vi "Get All Channels.vi"(7 "GUID (Default Channel)":string="03D3BB99-1485-13A6-561D1F898F032919", 8 "error in (no error)":errorcluster, 11 "Item Ref in":T1 format="%.0x") -> (0 "error out":errorcluster, 2 "Channels refs":T1[](array[typedef]) format="%.0x", 3 "Item Ref out":T1 format="%.0x")   [LabVIEW 2017, in "DSF Shared.lvlib"]
uses:
  DSF Shared.lvlib
  <vilib>/NI Veristand/Custom Device API/Custom Device Item Ref.ctl
  <vilib>/NI Veristand/Custom Device API/Custom Device API.lvlib
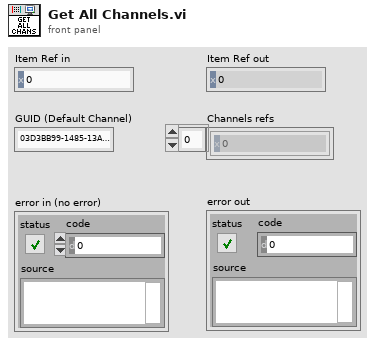
[diagram p1: front panel]
types:
  T1 = typedef "Custom Device API.lvlib/Custom Device Item Ref.ctl" = u64
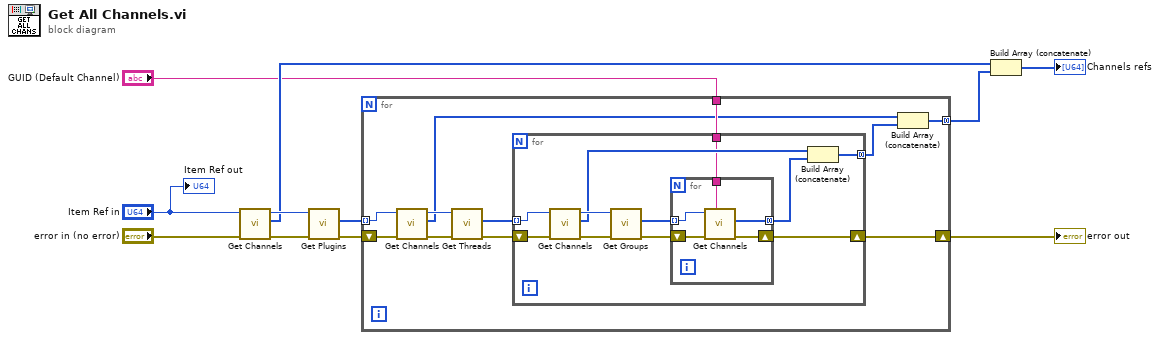
[diagram p0: block diagram]
diagram:
  n1 = call "Get Channels.vi"("error in (no error)"="error in (no error)", "Item Ref in"="Item Ref in") -> ("error out"=w6:errorcluster, "Channels refs"=w3:T1[], "Item Ref out"=w5:T1)  [unwired: 7 in]
  n2 = call "Get Plugins.vi"("error in (no error)"=w6, "Item Ref in"=w5) -> ("error out"=w11:errorcluster, "Plugin refs"=w10:T1[])  [unwired: 7 in, 1 out]
  n3 = for {
    tunnel: w10 -> [w19] mode=indexing
    tunnel: [w12] -> w8 mode=concatenating
    tunnel: "GUID (Default Channel)" -> [w21]
    shift-right: [w22] -> w2
    shift-left: w11 -> [w20]
    n4 = call "Get Channels.vi"("error in (no error)"=w20, "Item Ref in"=w19) -> ("error out"=w18:errorcluster, "Channels refs"=w13:T1[], "Item Ref out"=w17:T1)  [unwired: 7 in]
    n5 = call "Get Threads.vi"("error in (no error)"=w18, "Item Ref in"=w17) -> ("error out"=w16:errorcluster, "Plugin refs"=w15:T1[])  [unwired: 7 in, 1 out]
    n6 = for {
      shift-right: [w24] -> w22
      shift-left: w16 -> [w29]
      tunnel: w15 -> [w28] mode=indexing
      tunnel: [w31] -> w14 mode=concatenating
      tunnel: w21 -> [w23]
      n7 = call "Get Channels.vi"("error in (no error)"=w29, "Item Ref in"=w28) -> ("error out"=w27:errorcluster, "Channels refs"=w25:T1[], "Item Ref out"=w26:T1)  [unwired: 7 in]
      n8 = call "Get Groups.vi"("error in (no error)"=w27, "Plugin Ref in"=w26) -> ("error out"=w33:errorcluster, "Group refs"=w32:T1[])  [unwired: 7 in, 1 out]
      n9 = for {
        shift-right: [w36] -> w24
        shift-left: w33 -> [w38]
        tunnel: w32 -> [w37] mode=indexing
        tunnel: [w35] -> w30 mode=concatenating
        tunnel: w23 -> [w34]
        n10 = call "Get Channels.vi"("GUID (Default Channel)"=w34, "error in (no error)"=w38, "Item Ref in"=w37) -> ("error out"=w36:errorcluster, "Channels refs"=w35:T1[])  [unwired: 6 in, 1 out]
      }
      n11 = Build Array (concatenate)(w25, w30) -> (w31:T1[])
    }
    n12 = Build Array (concatenate)(w13, w14) -> (w12:T1[])
  }
  "error out" <- w2
  n13 = Build Array (concatenate)(w3, w8) -> (→"Channels refs":T1[])
  "Item Ref out" <- "Item Ref in"
